vi "Get Stop.vi"(5 "error in (no error)":errorcluster) -> (14 "Stop":bool, 19 "error out":errorcluster)   [LabVIEW 2013, in "Math.lvclass"]
uses:
  Math.lvclass
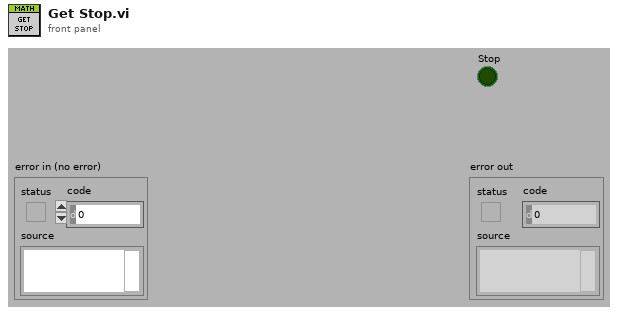
[diagram p1: front panel]
types:
  T1 = typedef "Math.lvclass/ClassAttributes.ctl" = cluster{"Stop":bool, "Rand":dbl}
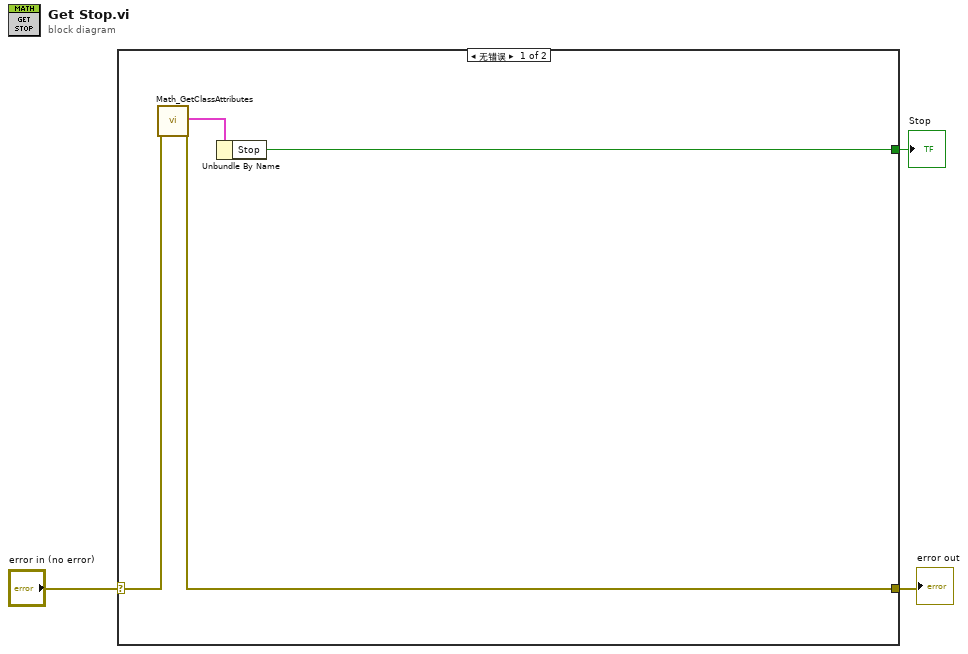
[diagram p0: block diagram]
diagram:
  n1 = case shown="无错误" "error in (no error)" {
    selector: "error in (no error)" -> [w7 w8]
    tunnel: [w6 w8] -> w2
    tunnel: [w4 _] -> w1
    frame No Error {
      n2 = call "Math_GetClassAttributes.vi"("error in (no error)"=w7) -> ("class attributes"=w5:T1, "error out"=w6:errorcluster)  [unwired: 15 in, 2 out]
      n3 = Unbundle By Name(w5) -> ("Stop"=w4:bool)
    }
    frame Error {
    }
  }
  "error out" <- w2
  "Stop" <- w1
